vi "FMA1600A General Send Receive.vi"(7 "Gas Type":T2, 8 "error in (no error)":errorcluster, 9 "Unit ID in":string, 10 "FMA1600A Commands":T3, 11 "VISA Refnum in":refnum<visa-resource-name>) -> (0 "error out":errorcluster, 1 "FMA1600A Gas Data":T1, 3 "VISA Refnum out":refnum<visa-resource-name>, 5 "Data Stream":string)   [LabVIEW 2016]
uses:
  Type Definitions/FMA1600A Commands.ctl
  Type Definitions/FMA1600A Gas Type.ctl
  Type Definitions/FMA1600A Data.ctl
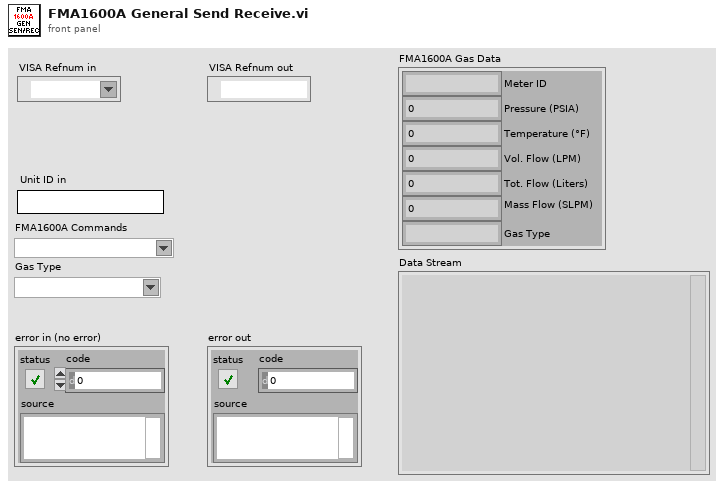
[diagram p1: front panel]
types:
  T1 = typedef "FMA1600A Data.ctl" = cluster{"Pressure (PSIA)":dbl, "Temperature (°F)":dbl, "Vol. Flow (LPM)":dbl, "Mass Flow (SLPM)":dbl, "Gas Type":string, "Tot. Flow (Liters)":dbl, "Meter ID":string}
  T2 = typedef "FMA1600A Gas Type.ctl" = string
  T3 = typedef "FMA1600A Commands.ctl" = string
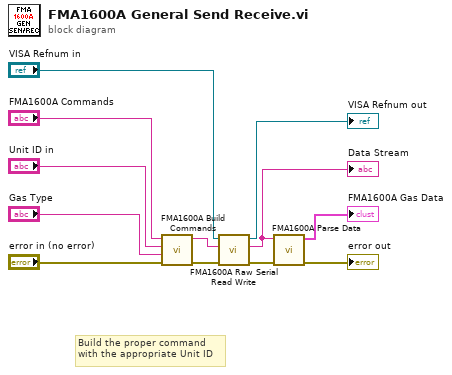
[diagram p0: block diagram]
diagram:
  # "Build the proper command\nwith the appropriate Unit ID"
  n1 = call "FMA1600A Build Commands.vi"("Error In"="error in (no error)", "Gas Type"="Gas Type", "Unit ID"="Unit ID in", "FMA1600A Commands"="FMA1600A Commands") -> ("Error Out"=w8:errorcluster, "Command Output"=w3:string)  [unwired: 6 in]
  n2 = call "FMA1600A Raw Serial Read Write.vi"("error in (no error)"=w8, "String"=w3, "VISA Refnum in"="VISA Refnum in") -> ("error out"=w9:errorcluster, "Data Stream"=w1:string, "VISA Refnum out"=→"VISA Refnum out":refnum<visa-resource-name>)  [unwired: 6 in]
  "Data Stream" <- w1
  n3 = call "FMA1600A Parse Data.vi"("Error In"=w9, "Raw FMA1600A Data"=w1) -> ("Error Out"=→"error out":errorcluster, "FMA1600A Gas Data"=→"FMA1600A Gas Data":T1)  [unwired: 7 in]
